vi "Construct Model Synchronously Requests Many Double Floats.vi"(9 "DBL Request Timeout (2000)":i32=2000) -> (1 "Results Notifier":refnum<notifier>, 3 "ModelSynchronouslyRequestsManyDoubleFloats Out":refnum<class "ModelSynchronouslyRequestsManyDoubleFloats.lvclass">)   [LabVIEW 2017, in "ModelSynchronouslyRequestsManyDoubleFloats.lvclass"]
uses:
  ModelSynchronouslyRequestsManyDoubleFloats.lvclass
  ModelSynchronouslyRequestsManyDoubleFloats.lvclass/ModelSynchronouslyRequestsManyDoubleFloats.ctl
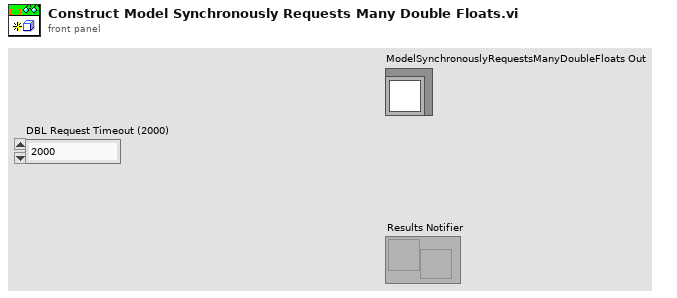
[diagram p1: front panel]
types:
  T1 = cluster{"Received Value":dbl, "Timed Out?":bool, "Sync Request Error":errorcluster}[]
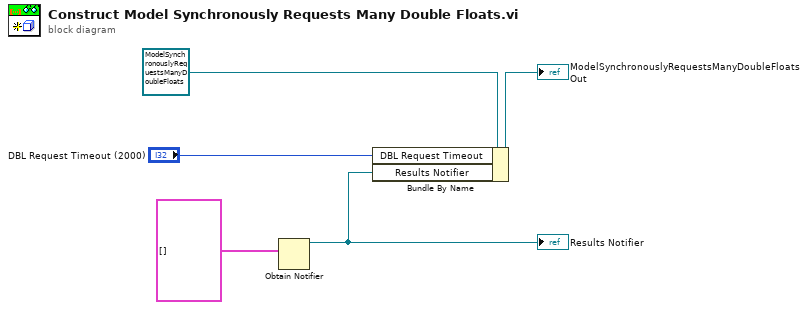
[diagram p0: block diagram]
diagram:
  n1 = Obtain Notifier(notification data type=T1 []) -> (notifier out=w1:refnum<notifier>)  [unwired: 3 in, 2 out]
  "Results Notifier" <- w1
  n2 = Bundle By Name(cluster=refnum<class "ModelSynchronouslyRequestsManyDoubleFloats.lvclass"> refnum ("ModelLeaksStateAfterLaunch in"), "DBL Request Timeout"="DBL Request Timeout (2000)", "Results Notifier"=w1) -> (→"ModelSynchronouslyRequestsManyDoubleFloats Out":refnum<class "ModelSynchronouslyRequestsManyDoubleFloats.lvclass">)
